vi "文件名.vi"(8 "第n个文件":i32, 9 "文件类型":i32, 11 "文件夹路径":path caption="路径") -> (2 "添加的路径":path)   [LabVIEW 2018]
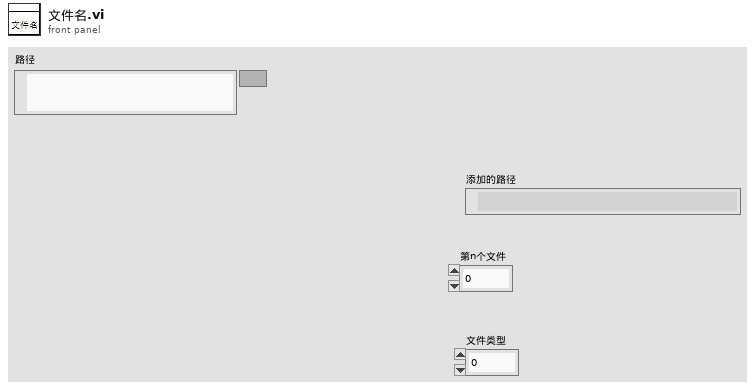
[diagram p1: front panel]
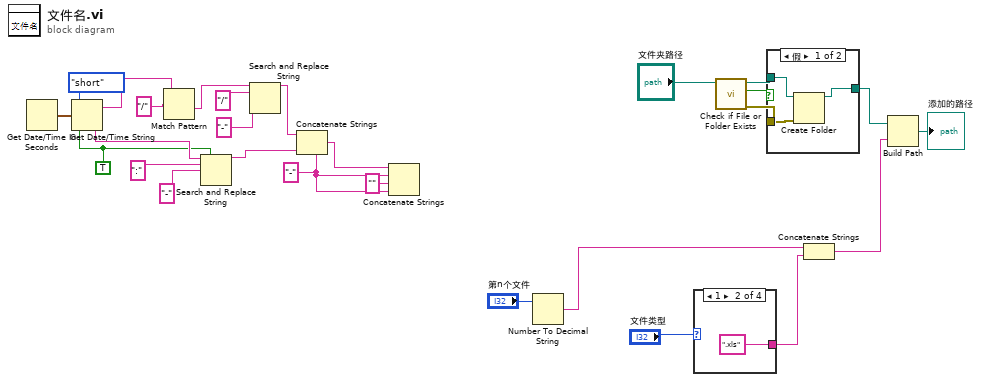
[diagram p0: block diagram]
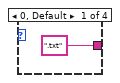
[diagram p2: hidden frame]
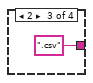
[diagram p3: hidden frame]
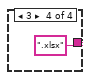
[diagram p4: hidden frame]
diagram:
  w6 = TRUE ("需要秒？(F)")
  w19 = "-" ("字符串")
  n1 = Get Date/Time In Seconds() -> (seconds since 1Jan1904=w27:timestamp)
  n2 = Get Date/Time String(date format (0)=enum16{"short", "long", "abbreviated"}."short" ("日期格式(0)"), seconds (now)=w27, want seconds? (F)=w6) -> (date string=w25:string, time string=w14:string)
  n3 = Match Pattern(string=w25, regular expression="/" ("正则表达式")) -> (after substring=w18:string)  [unwired: 1 in, 3 out]
  n4 = Search and Replace String(replace all?=w6, input string=w14, search string=":" ("搜索字符串"), replace string="-" ("替换字符串(\"\")")) -> (result string=w11:string)  [unwired: 4 in, 3 out]
  n5 = Search and Replace String(input string=w18, search string="/" ("搜索字符串"), replace string="-" ("替换字符串(\"\")")) -> (result string=w16:string)  [unwired: 5 in, 3 out]
  n6 = Concatenate Strings(w16, w19, w11) -> (w21:string)
  n7 = Concatenate Strings(w21, w19, "" ("字符串"), w19) -> ()  [unwired: 1 out]
  n8 = Number To Decimal String(number="第n个文件") -> (decimal integer string=w2:string)  [unwired: 1 in]
  n9 = case shown="1" "文件类型" {
    tunnel: [".txt" ".xls" ".csv" ".xlsx"] -> w5
    frame 0, Default {
    }
    frame 1 {
    }
    frame 2 {
    }
    frame 3 {
    }
  }
  n10 = call <vilib>:"Check if File or Folder Exists.vi"("path"="文件夹路径") -> ("error out"=w7:errorcluster, "file or folder exists?"=w10:bool, "dup path"=w8:path)  [unwired: 8 in]
  n11 = case shown="假" w10 {
    tunnel: [w34 w35] -> w9
    tunnel: w8 -> [w33 w35]
    tunnel: w7 -> [w32 _]
    frame False {
      n12 = Create Folder(path (use dialog)=w33, error in=w32) -> (created path=w34:path)  [unwired: 1 in, 2 out]
    }
    frame True {
    }
  }
  n13 = Concatenate Strings(w2, w5) -> (w22:string)
  n14 = Build Path(base path=w9, name or relative path=w22) -> (appended path=→"添加的路径":path)
